vi "Configure Trigger (UDTV).vi"(0 "VISA resource name":refnum<visa-resource-name>, 1 "Sync Pulse Time (3.178E-5 s)":dbl=3.178e-05, 5 "Number of Events (1)":i32=1, 7 "Enable Horizontal Sync Mode (F: Disable)":bool, 9 "Sync Pulse Polarity (0: Negative)":i32(ring) items=["Negative", "Positive"], 11 "error in (no error)":errorcluster, 12 "Minimum Pulse Width (2.6E-5 s)":dbl=2.6e-05) -> (4 "VISA resource name out":refnum<visa-resource-name>, 15 "error out":errorcluster)   [LabVIEW 2020, in "Agilent 90000 Series.lvlib"]
doc: "Configure user-defined TV trigger parameters."
uses:
  Agilent 90000 Series.lvlib
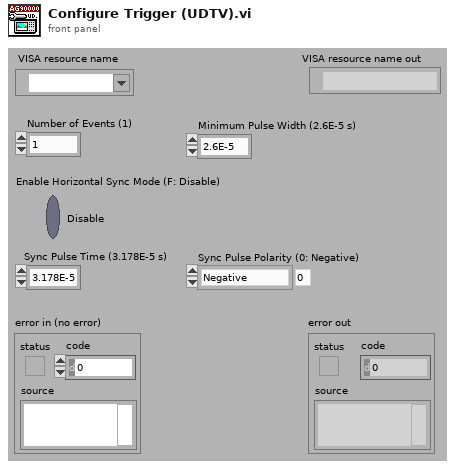
[diagram p1: front panel]
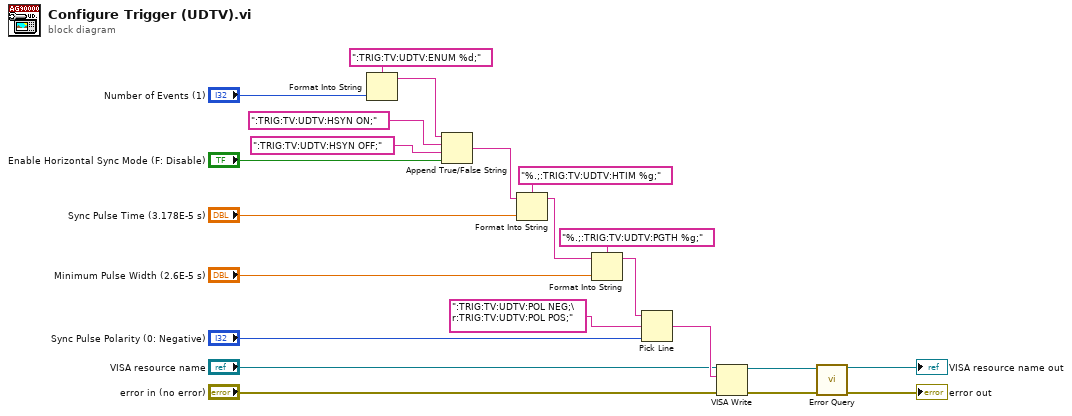
[diagram p0: block diagram]
diagram:
  n1 = Format Into String(format string=":TRIG:TV:UDTV:ENUM %d;", "Number of Events (1)") -> (resulting string=w20:string)  [unwired: 2 in, 1 out]
  n2 = Append True/False String(1:"Enable Horizontal Sync Mode (F: Disable)", 2:":TRIG:TV:UDTV:HSYN OFF;", 3:":TRIG:TV:UDTV:HSYN ON;", 4:w20) -> (0:w16:string)
  n3 = Format Into String(format string="%.;:TRIG:TV:UDTV:HTIM %g;", initial string=w16, "Sync Pulse Time (3.178E-5 s)") -> (resulting string=w13:string)  [unwired: 1 in, 1 out]
  n4 = Format Into String(format string="%.;:TRIG:TV:UDTV:PGTH %g;", initial string=w13, "Minimum Pulse Width (2.6E-5 s)") -> (resulting string=w10:string)  [unwired: 1 in, 1 out]
  n5 = Pick Line(string ("")=w10, multi-line string=":TRIG:TV:UDTV:POL NEG;\r:TRIG:TV:UDTV:POL POS;", line index="Sync Pulse Polarity (0: Negative)") -> (output string=w7:string)
  n6 = VISA Write(VISA resource name="VISA resource name", write buffer=w7, error in (no error)="error in (no error)") -> (VISA resource name out=w4:refnum<visa-resource-name>, error out=w3:errorcluster)  [unwired: 1 out]
  n7 = call "Error Query.vi"("error in (no error)"=w3, "VISA resource name"=w4) -> ("error out"=→"error out":errorcluster, "VISA resource name out"=→"VISA resource name out":refnum<visa-resource-name>)  [unwired: 8 out]
